vi "ModeCheck.vi"(4 "Row Span (all)":i32=-1, 6 "Start Row (first, DISAB only)":i32=-1, 8 "error in (no error)":errorcluster, 9 "mode col. index":i32=2, 10 "Col Array in":refnum<class "Column.lvclass">[](array[class]), 11 "Table Ref in":refnum<vi>) -> (0 "error out":errorcluster, 3 "Table Ref out":refnum<vi>)   [LabVIEW 2013]
doc: "Ensure that Slave device rows are not editable when row is Continue/Loop/End Loop, as read from the column in Table Ref at the Mode Col index. To speed up execution of slow table coloring, this VI can be used in two modes: (1) Start Row < 0 -- DISABLE only (only safe to use if the table has been reformatted!) (2) StartRow >=0 -- ENABLE/DISABLE for all rows in span (negative span indicates all rows)\nWhen Start and Span are not provided all rows are set with (1) above."
uses:
  ColumnVIs/Column/Column.lvclass
  ColumnVIs/ModeCol/ModeCol.lvclass
  <vilib>/Utility/miscctls.llb/LVRowAndColumnTypeDef.ctl
panel:
  out "DISAB only?":bool
  out "all?":bool
  # "Possibly add input (integer array) to denote start and span of rows to check."
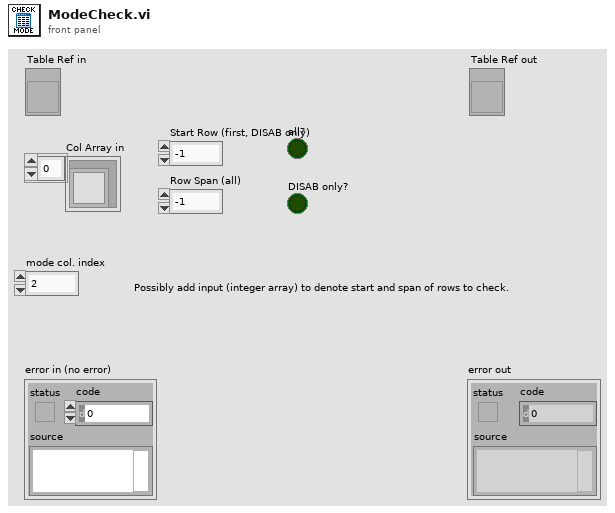
[diagram p1: front panel]
types:
  T1 = typedef "LVRowAndColumnTypeDef.ctl" = cluster{"Row":i32, "Column":i32}
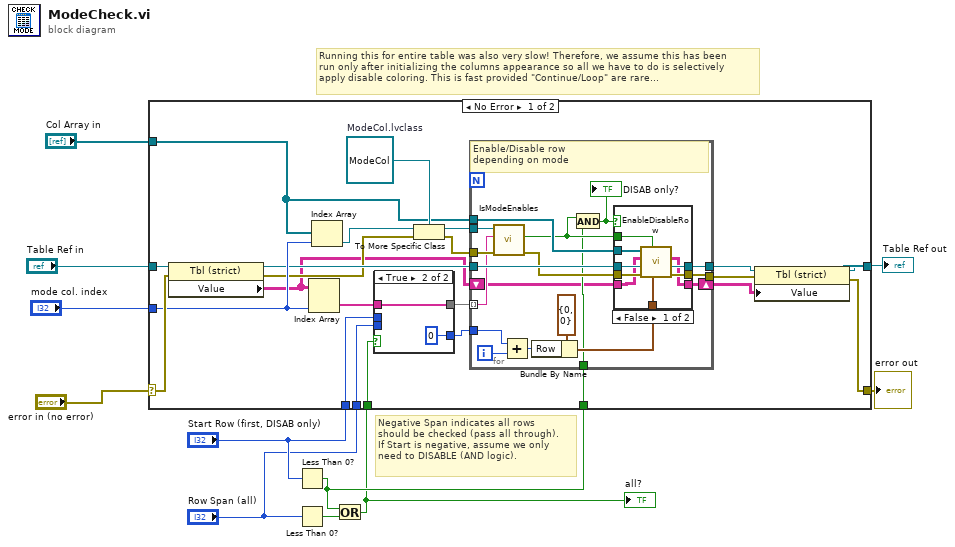
[diagram p0: block diagram]
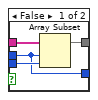
[diagram p2: hidden frame]
diagram:
  # "Negative Span indicates all rows\nshould be checked (pass all through).\nIf Start is negative, assume we only \nneed to DISABLE (AND logic)."
  # "Running this for entire table was also very slow! Therefore, we assume this has been\nrun only after initializing the columns appearance so all we have to do is selectively\napply disable coloring. This is fast provided \"Continue/Loop\" are rare..."
  n1 = Less Than 0?(x="Start Row (first, DISAB only)") -> (x < 0?=w3:bool)
  n2 = Less Than 0?(x="Row Span (all)") -> (x < 0?=w2:bool)
  n3 = Or(x=w3, y=w2) -> (x .or. y?=w1:bool)
  "all?" <- w1
  n4 = case shown="No Error" "error in (no error)" {
    selector: "error in (no error)" -> [w33 w72]
    tunnel: [w13 w72] -> w10
    tunnel: "Table Ref in" -> [w34 w71]
    tunnel: [w15 w71] -> w8
    tunnel: "mode col. index" -> [w32 _]
    tunnel: "Col Array in" -> [w25 _]
    tunnel: "Start Row (first, DISAB only)" -> [w21 _]
    tunnel: "Row Span (all)" -> [w23 _]
    tunnel: w3 -> [w20 _]
    tunnel: w1 -> [w19 _]
    frame No Error {
      w28 = refnum<class "ModeCol.lvclass"> refnum  # ModeCol.lvclass
      n5 = property class="Tbl (strict)"(reference=w34, error in=w33) -> (reference out=w31:refnum<vi>, error out=w26:errorcluster, "Value"=w17:string[][])
      n6 = Index Array(array=w17, index (col)=w32) -> (element=w24:string[])  [unwired: 1 in]
      n7 = Index Array(array=w25, index=w32) -> (element=w29:refnum<class "Column.lvclass">)
      n8 = case shown="True" w19 {
        tunnel: w24 -> [w38 w40]
        tunnel: w23 -> [w37 _]
        tunnel: [w36 w40] -> w22
        tunnel: w21 -> [w35 _]
        tunnel: [w35 0 ("Start Row (first)")] -> w18
        frame False {
          n9 = Array Subset(array=w38, index=w35, length=w37) -> (w36:string[])
        }
        frame True {
        }
      }
      n10 = To More Specific Class(target class=w28, reference=w29, error in=w26) -> (specific class reference=w27:refnum<class "ModeCol.lvclass">, error out=w30:errorcluster)
      n11 = for {
        tunnel: w30 -> [w52]
        tunnel: [w56] -> w14
        tunnel: w22 -> [w51] mode=indexing
        tunnel: w27 -> [w50]
        tunnel: w25 -> [w49]
        tunnel: w31 -> [w58]
        tunnel: [w57] -> w16
        tunnel: w20 -> [w45]
        tunnel: w18 -> [w44]
        shift-right: [w41] -> w12
        shift-left: w17 -> [w42]
        i -> [w43]
        # "Enable/Disable row \ndepending on mode"
        n12 = call "IsModeEnables.vi"("error in (no error)"=w52, "Mode value"=w51, "ModeCol in"=w50) -> ("error out"=w53:errorcluster, "Disable / Enable"=w46:bool)  [unwired: 6 in, 1 out]
        n13 = Add(x=w44, y=w43) -> (x+y=w48:i32)
        n14 = Bundle By Name(cluster=T1 {"Row"=0, "Column"=0} ("Cell Position"), "Row"=w48) -> (w55:T1)
        n15 = And(x=w46, y=w45) -> (x .and. y?=w47:bool)
        "DISAB only?" <- w47
        n16 = case shown="False" w47 {
          tunnel: w58 -> [w67 w70]
          tunnel: [w66 w70] -> w57
          tunnel: [w65 w69] -> w56
          tunnel: w55 -> [w64 _]
          tunnel: w53 -> [w63 w69]
          tunnel: w49 -> [w62 _]
          tunnel: w46 -> [w61 _]
          tunnel: w42 -> [w60 w68]
          tunnel: [w59 w68] -> w41
          frame False {
            n17 = call "EnableDisableRow.vi"("Cell Position"=w64, "Disable / Enable"=w61, "error in (no error)"=w63, "Table CtlRef In"=w67, "Table Data in"=w60, "Col Array in"=w62) -> ("error out"=w65:errorcluster, "Table CtlRef Out"=w66:refnum<vi>, "Table Data out"=w59:string[][])  [unwired: 3 in]
          }
          frame True {
          }
        }
      }
      n18 = property class="Tbl (strict)"(reference=w16, error in=w14, "Value"=w12) -> (reference out=w15:refnum<vi>, error out=w13:errorcluster)
    }
    frame Error {
    }
  }
  "error out" <- w10
  "Table Ref out" <- w8
